vi "Emballage_BDD_afficheInfoCmdInterne.vi"(8 "Error in":errorcluster caption="Error in (no error)", 10 "nbr de pièce":i32 caption="Nombre de pièces:", 11 "CMD interne":string caption="N° de commande interne:") -> (0 "Error out":errorcluster)   [LabVIEW 2020]
panel:
  in  "Bouton OK":bool
  # "Votre commande interne est terminée!"
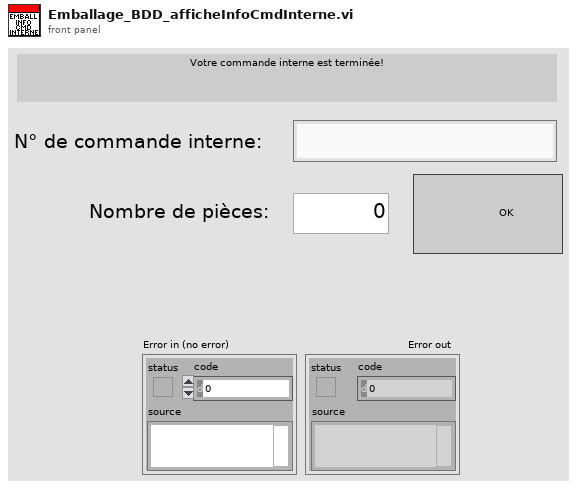
[diagram p1: front panel]
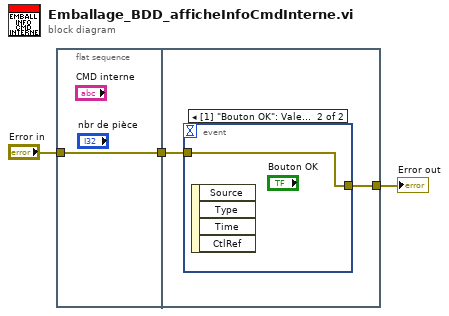
[diagram p0: block diagram]
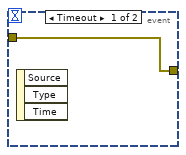
[diagram p2: hidden frame]
diagram:
  n1 = flat-sequence {
    tunnel: "Error in" -> [w4]
    tunnel: [w4] -> w1
    tunnel: [w5] -> w2
    tunnel: w1 -> [w6]
    frame #0 {
    }
    frame #1 {
      n2 = event shown="[1] \"Bouton OK\": Valeur changée" {
        selector: _ -> [_ _]
        dyn-events: _ -> [_ _]
        timeout: _ -> [_ _]
        tunnel: w6 -> [w7 w8]
        tunnel: [w7 w8] -> w5
        event Timeout {
          n3 = event-data() -> ()  [unwired: 1 in, 3 out]
        }
        event "Bouton OK": Value Change {
          n4 = event-data() -> ()  [unwired: 1 in, 4 out]
        }
      }
    }
  }
  "Error out" <- w2
